vi "GenericDriveWriteMulti.vi"(5 "Channel Description":T3={"Channel Name"="", "Vel. Default"=5.0, "Acc. Default"=5.0, "Vel. Max"=5.0, "Vel. Min"=5.0, "Acc. Max"=5.0, "Acc. Min"=5.0, "Pulses/unit"=0.0, "Address"=0, "Pulse Offset"=0, "Pos Tolerance"=0.0, "Pulses/rev"=0.0, "Backlash/Eng units"=0.0, "Current Pos"=0.0, "Ch Status"=enum."Active", "Port Name"="", "Axis Transform mode"="", "Metadata Ch Name"="", "Type"=enum."MCode", "De Power Motor"=enum."FALSE", "ConfigString"=""} {"Current Pos" format="%.2f"; "Backlash/Eng units" format="%.2f"; "Pulses/rev" format="%.2f"; "Pos Tolerance" format="%.2f"; "Pulses/unit" format="%.2f"; "Acc. Min" format="%.2f"; "Acc. Max" format="%.2f"; "Vel. Min" format="%.2f"; "Vel. Max" format="%.2f"; "Acc. Default" format="%.2f"; "Vel. Default" format="%.2f"}, 6 "Array Constant":T2(array[cluster])=[{"GenericDriveCommand"="DePowerMotor", "Numeric Value"=0.0}, {"GenericDriveCommand"="DePowerMotor", "Numeric Value"=0.0}, {"GenericDriveCommand"="DePowerMotor", "Numeric Value"=0.0}] {"Numeric Value" format="%.2f"}) -> (0 "Error Description":string)   [LabVIEW 2022 SP3]
uses:
  DriveProperties.ctl
  Traverse Type.ctl
  GenericDriveCommand.ctl
  Dynamixel/Sub Vis/Dynamixel Commands.ctl
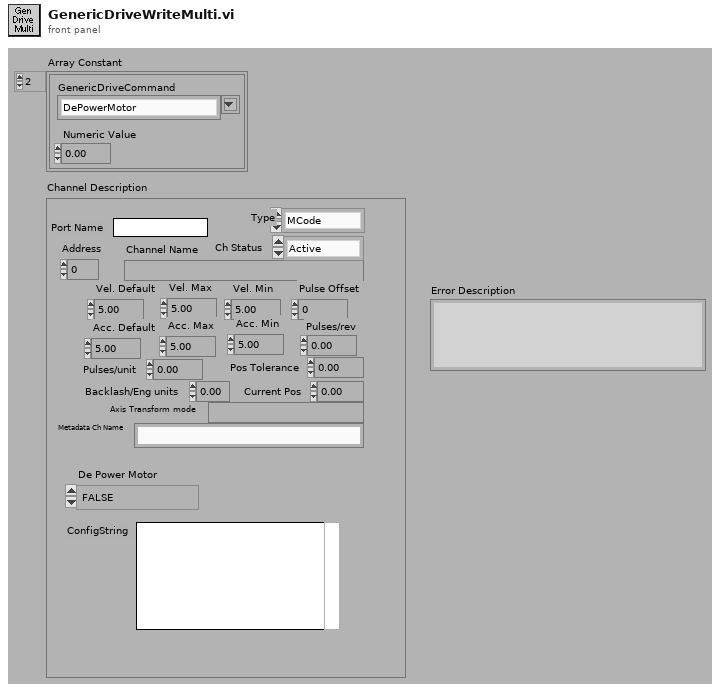
[diagram p1: front panel]
types:
  T1 = typedef "GenericDriveCommand.ctl" = string
  T2 = cluster{"GenericDriveCommand":T1, "Numeric Value":dbl}[]
  T3 = typedef "DriveProperties.ctl" = cluster{"Channel Name":string, "Vel. Default":sgl, "Acc. Default":sgl, "Vel. Max":sgl, "Vel. Min":sgl, "Acc. Max":sgl, "Acc. Min":sgl, "Pulses/unit":sgl, "Address":u8, "Pulse Offset":i32, "Pos Tolerance":sgl, "Pulses/rev":sgl, "Backlash/Eng units":sgl, "Current Pos":sgl, "Ch Status":enum16{"Active", "Offline", "Simulate"}, "Port Name":string, "Axis Transform mode":string, "Metadata Ch Name":string, "Type":T4, "De Power Motor":enum16{"TRUE", "FALSE"}, "ConfigString":string}
  T4 = typedef "Traverse Type.ctl" = enum16{"MCode", "Dynamixel"}
  T5 = typedef "Dynamixel Commands.ctl" = enum16{"Torque Enable", "Present Position", "Threshold", "Max Position Limit", "Acceleration Profile", "Velocity Profile", "Goal Position", "Position Proportional Gain", "Position Integral Gain", "Position Differential Gain ", "Shutdown", "Write Operating Mode", "Read Operating Mode"}
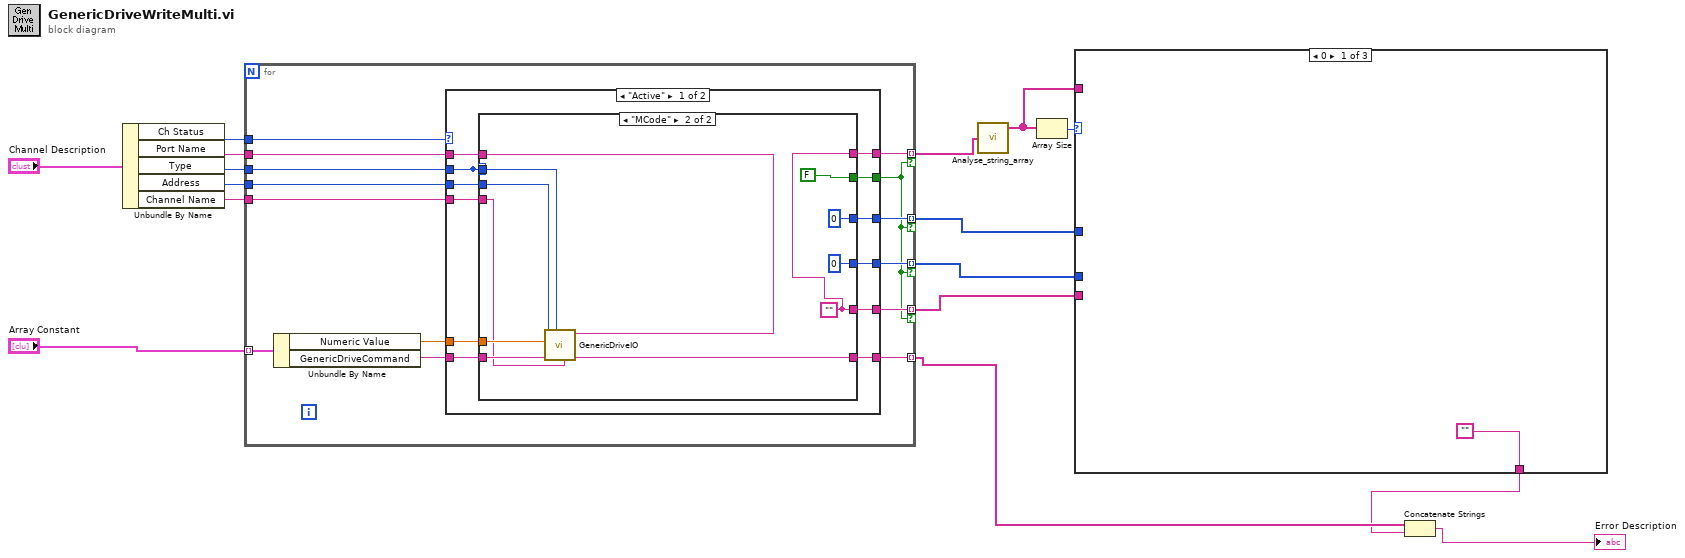
[diagram p0: block diagram]
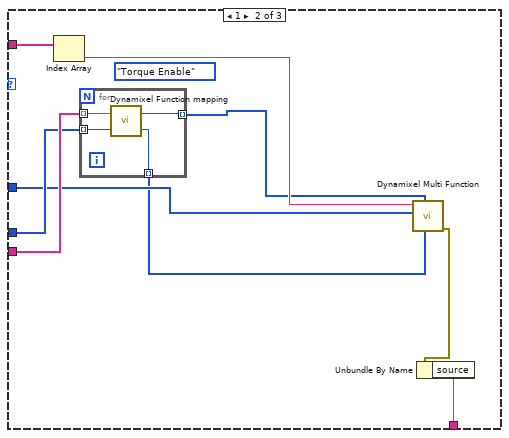
[diagram p2: hidden frame]
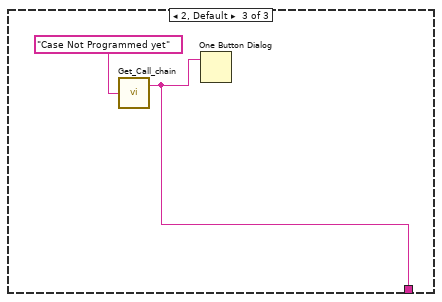
[diagram p3: hidden frame]
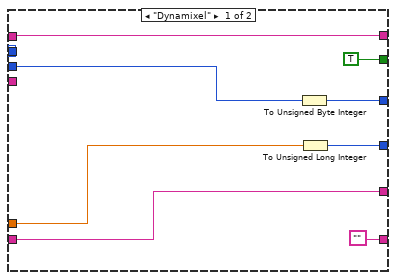
[diagram p4: hidden frame]
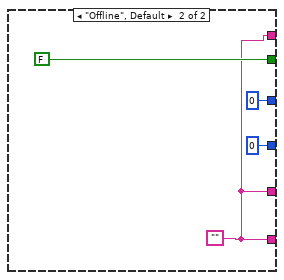
[diagram p5: hidden frame]
diagram:
  n1 = Unbundle By Name("Channel Description") -> ("Ch Status"=w15:enum16{"Active", "Offline", "Simulate"}, "Port Name"=w14:string, "Type"=w13:T4, "Address"=w12:u8, "Channel Name"=w11:string)
  n2 = for {
    tunnel: "Array Constant" -> [w30] mode=indexing
    tunnel: w15 -> [w29]
    tunnel: w14 -> [w28]
    tunnel: w13 -> [w27]
    tunnel: w12 -> [w26]
    tunnel: w11 -> [w23]
    tunnel: [w22] -> w3 mode=indexing
    tunnel: [w21] -> w6 mode=indexing if=w17
    tunnel: [w20] -> w4 mode=indexing if=w17
    tunnel: [w19] -> w5 mode=indexing if=w17
    tunnel: [w18] -> w9 mode=indexing if=w17
    n3 = Unbundle By Name(w30) -> ("Numeric Value"=w25:dbl, "GenericDriveCommand"=w24:T1)
    n4 = case shown="\"Active\"" w29 {
      tunnel: w28 -> [w42 _]
      tunnel: w27 -> [w36 _]
      tunnel: w26 -> [w41 _]
      tunnel: w25 -> [w40 _]
      tunnel: w24 -> [w39 _]
      tunnel: w23 -> [w38 _]
      tunnel: [w37 w62] -> w22
      tunnel: [w35 FALSE] -> w17
      tunnel: [w34 u8 0] -> w21
      tunnel: [w33 w62] -> w20
      tunnel: [w32 u32 0] -> w19
      tunnel: [w31 w62] -> w18
      frame "Active" {
        n5 = case shown="\"MCode\"" w36 {
          tunnel: w42 -> [w43 w55]
          tunnel: w36 -> [_ w61]
          tunnel: w41 -> [w48 w60]
          tunnel: w40 -> [w45 w59]
          tunnel: w39 -> [w46 w58]
          tunnel: w38 -> [_ w57]
          tunnel: ["" w56] -> w37
          tunnel: [TRUE FALSE] -> w35
          tunnel: [w47 u8 0] -> w34
          tunnel: [w46 w51] -> w33
          tunnel: [w44 u32 0] -> w32
          tunnel: [w43 w51] -> w31
          frame "Dynamixel" {
            n6 = To Unsigned Byte Integer(number=w48) -> (unsigned 8bit integer=w47:u8)
            n7 = To Unsigned Long Integer(number=w45) -> (unsigned 32bit integer=w44:u32)
          }
          frame "MCode" {
            w51 = ""
            n8 = call "GenericDriveIO.vi"("GenericDriveCommand"=w58, "Channel Name"=w57, "Numeric Value"=w59, "Address"=w60, "Type"=w61, "Port Name"=w55) -> ("Error Description"=w56:string)  [unwired: 1 in, 4 out]
          }
        }
      }
      frame "Offline", Default {
        w62 = ""
      }
    }
  }
  n9 = call "Analyse_string_array.vi"("String array"=w9) -> ("Unique strings"=w7:string[])  [unwired: 1 in, 1 out]
  n10 = Array Size(array=w7) -> (size(s)=w8:i32)
  n11 = case shown="0" w8 {
    tunnel: w7 -> [_ w75 _]
    tunnel: w6 -> [_ w70 _]
    tunnel: w5 -> [_ w72 _]
    tunnel: w4 -> [_ w73 _]
    tunnel: ["" w67 w80] -> w2
    frame 0 {
    }
    frame 1 {
      (unwired) Dynamixel_Commands."Torque Enable" ("Function")
      n12 = Index Array(array=w75) -> (element=w74:string)  [unwired: 1 in]
      n13 = for {
        tunnel: w73 -> [w79] mode=indexing
        tunnel: [w78] -> w71 mode=indexing
        tunnel: w72 -> [w77] mode=indexing
        tunnel: [w76] -> w69 mode=indexing
        n14 = call "Dynamixel Function mapping.vi"("data In"=w77, "GenericDriveCommand"=w79) -> ("data Out"=w76:u32, "Function"=w78:T5)
      }
      n15 = call "Dynamixel Multi Function.vi"("Data Array"=w69, "Function Array"=w71, "Motor ID"=w70, "Com port"=w74) -> ("error out"=w68:errorcluster)  [unwired: 6 in, 1 out]
      n16 = Unbundle By Name(w68) -> ("source"=w67:string)
    }
    frame 2, Default {
      n17 = call "Get_Call_chain.vi"("Message"="Case Not Programmed yet" ("message")) -> ("Output String"=w80:string)  [unwired: 1 out]
      n18 = One Button Dialog(message=w80) -> ()  [unwired: 1 in, 1 out]
    }
  }
  n19 = Concatenate Strings(w3, w2) -> (→"Error Description":string)
